vi "Generate sine.vi"(5 "input dt":dbl, 7 "samples":i32, 11 "Current treatment":T1) -> (1 "vel":dbl[](array[numeric]), 2 "pos":dbl[](array[numeric]), 3 "Treatment out":T1)   [LabVIEW 2012]
uses:
  Treatment.ctl
  Treatment type.ctl
  <vilib>/Analysis/NI_AALBase.lvlib
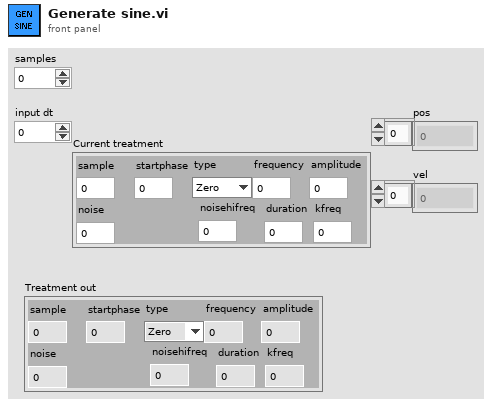
[diagram p1: front panel]
types:
  T1 = typedef "Treatment.ctl" = cluster{"sample":dbl, "startphase":dbl, "type":T2, "frequency":dbl, "amplitude":dbl, "noise":dbl, "duration":dbl, "kfreq":dbl, "noisehifreq":dbl}
  T2 = typedef "Treatment type.ctl" = enum16{"Zero", "Sine", "Frequency sweep"}
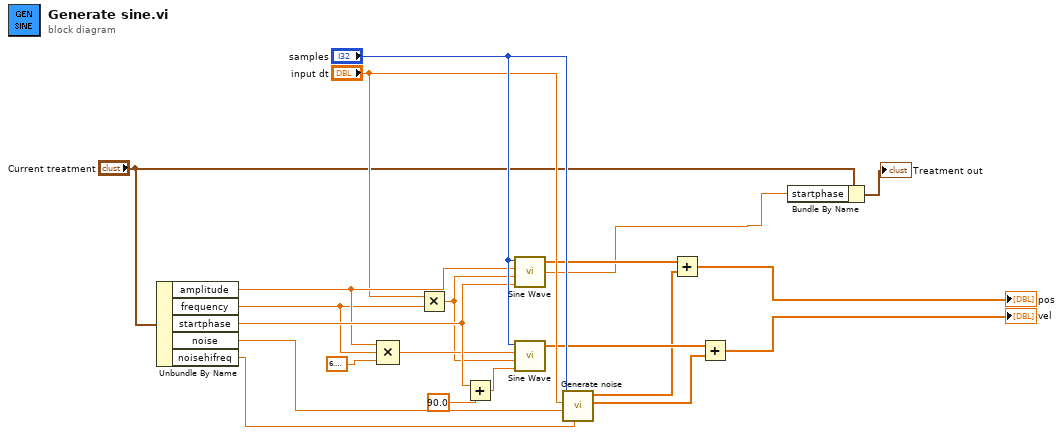
[diagram p0: block diagram]
diagram:
  n1 = Unbundle By Name("Current treatment") -> ("amplitude"=w18:dbl, "frequency"=w14:dbl, "startphase"=w19:dbl, "noise"=w21:dbl, "noisehifreq"=w1:dbl)
  n2 = Compound Arithmetic op=MULTIPLY(w18, w14, 6.283185307179586) -> (w12:dbl)
  n3 = Multiply(x="input dt", y=w14) -> (x*y=w10:dbl)
  n4 = Add(x=w19, y=90.0) -> (x+y=w8:dbl)
  n5 = call <vilib>:"Sine Wave.vi"("samples"="samples", "amplitude"=w18, "frequency"=w10, "phase in"=w19) -> ("sine wave"=w9:dbl[], "phase out"=w3:dbl)  [unwired: 1 in, 1 out]
  n6 = call <vilib>:"Sine Wave.vi"("samples"="samples", "amplitude"=w12, "frequency"=w10, "phase in"=w8) -> ("sine wave"=w11:dbl[])  [unwired: 1 in, 2 out]
  n7 = call "Generate noise.vi"("noisehifreq"=w1, "noise std"=w21, "input dt"="input dt", "samples"="samples") -> ("noise deriv"=w5:dbl[], "noise"=w6:dbl[])  [unwired: 6 in]
  n8 = Add(x=w9, y=w6) -> (x+y=→"pos":dbl[])
  n9 = Add(x=w11, y=w5) -> (x+y=→"vel":dbl[])
  n10 = Bundle By Name(cluster="Current treatment", "startphase"=w3) -> (→"Treatment out":T1)
